vi "record_pressures.vi"() -> ()   [LabVIEW 2016]
uses:
  Globals/PressuresGlobal.vi
panel:
  in  "Set Points":dbl[](array[numeric])=[0.1, 0.2, 0.3, 0.4, 0.5, 0.6, 0.7, 0.8, 0.9]
  in  "stop":bool
  in  "Use Control":bool
  out "Pressure Array":dbl[][](array[numeric])
  in  "Use This Pressure":bool
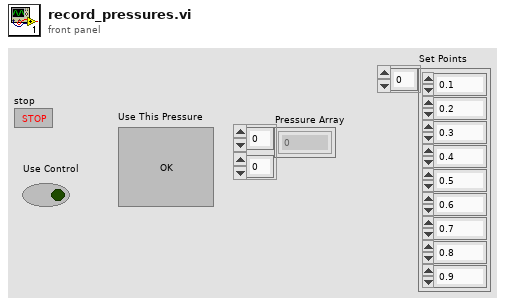
[diagram p1: front panel]
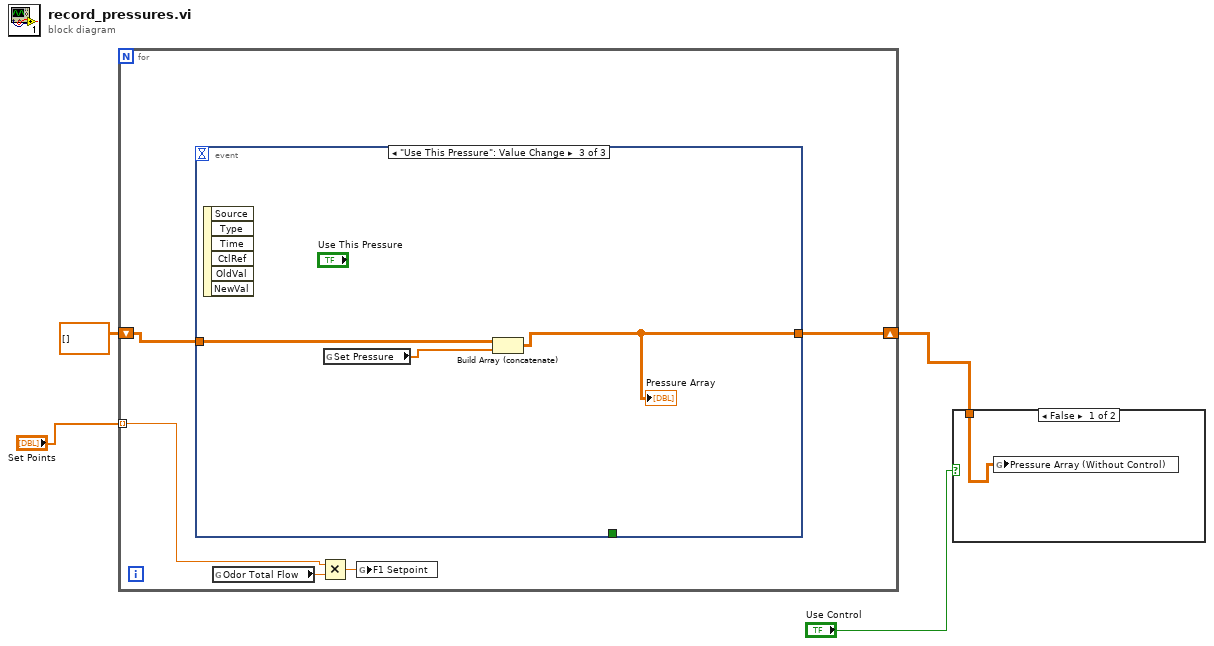
[diagram p0: block diagram]
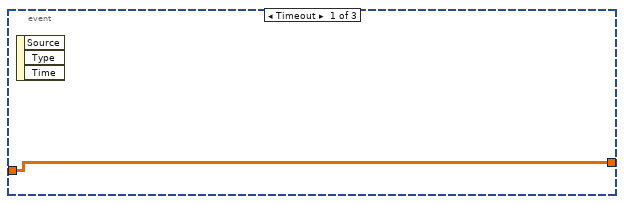
[diagram p2: hidden frame]
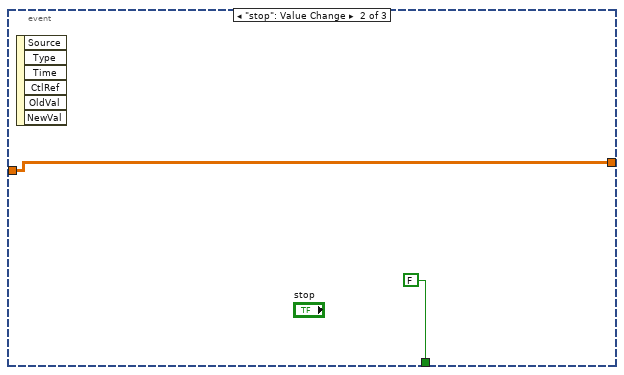
[diagram p3: hidden frame]
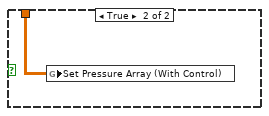
[diagram p4: hidden frame]
diagram:
  n1 = for {
    shift-right: [w9] -> w2
    shift-left: dbl[][] [] -> [w8]
    tunnel: "Set Points" -> [w5] mode=indexing
    n2 = event shown="[2] \"Use This Pressure\": Value Change" {
      selector: _ -> [_ _ _]
      dyn-events: _ -> [_ _ _]
      timeout: _ -> [_ _ _]
      tunnel: [w10 w12 w13] -> w9
      tunnel: w8 -> [w10 w12 w14]
      tunnel: [_ FALSE _] -> _
      event Timeout {
        n3 = event-data() -> ()  [unwired: 1 in, 3 out]
      }
      event "stop": Value Change {
        n4 = event-data() -> ()  [unwired: 1 in, 6 out]
      }
      event "Use This Pressure": Value Change {
        n5 = event-data() -> ()  [unwired: 1 in, 6 out]
        n6 = global read "PressuresGlobal.vi" "Set Pressure"() -> (w15:dbl[])
        n7 = Build Array (concatenate)(w14, w15) -> (w13:dbl[][])
        "Pressure Array" <- w13
      }
    }
    n8 = global read "PressuresGlobal.vi" "Odor Total Flow"() -> (w6:dbl)
    n9 = Multiply(x=w5, y=w6) -> (x*y=w7:dbl)
    n10 = global write "PressuresGlobal.vi" "F1 Setpoint"(w7) -> ()
  }
  n11 = case shown="False" "Use Control" {
    tunnel: w2 -> [w16 w17]
    frame False {
      n12 = global write "PressuresGlobal.vi" "Pressure Array (Without Control)"(w16) -> ()
    }
    frame True {
      n13 = global write "PressuresGlobal.vi" "Set Pressure Array (With Control)"(w17) -> ()
    }
  }
